vi "CreateIlluminationMask.vi"(7 "# Pixels":u16, 8 "error in (no error)":errorcluster, 9 "Image trig index":u16[](array[numeric]), 10 "Time at P_f":u32[](array[numeric]), 11 "Final step, n":u16[](array[numeric])) -> (0 "error out":errorcluster, 1 "Image trig index OUT":u16[](array[numeric]), 2 "Time at P_f 2":u16[](array[numeric]), 3 "Final step OUT":u16[](array[numeric]), 4 "Time at P_f 2D":u16[][](array[numeric]), 5 "Final step 2D":u16[][](array[numeric]))   [LabVIEW 2016]
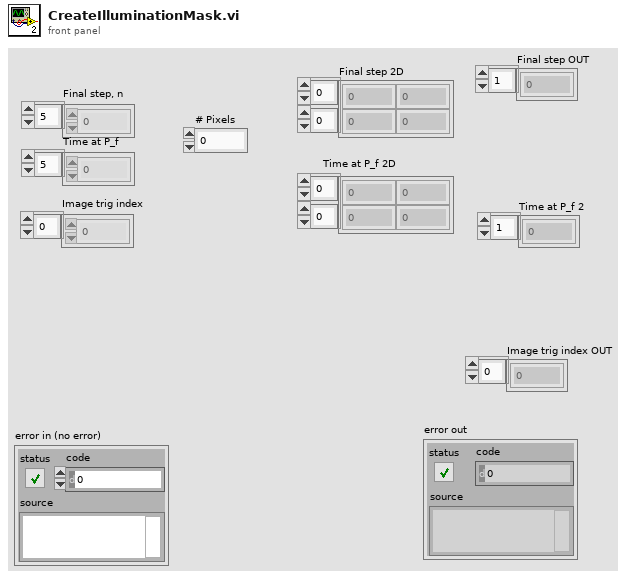
[diagram p1: front panel]
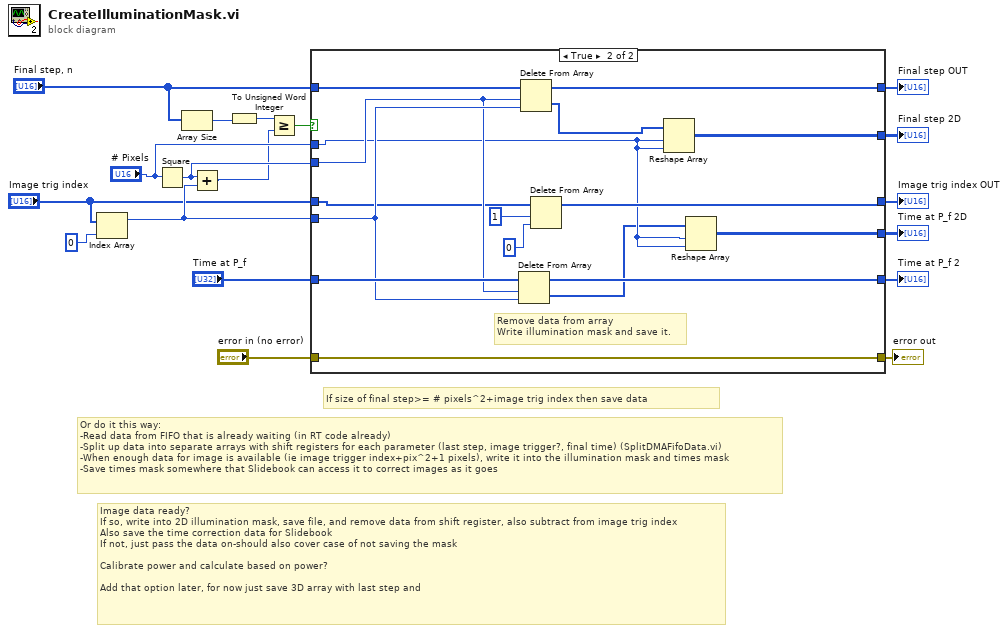
[diagram p0: block diagram]
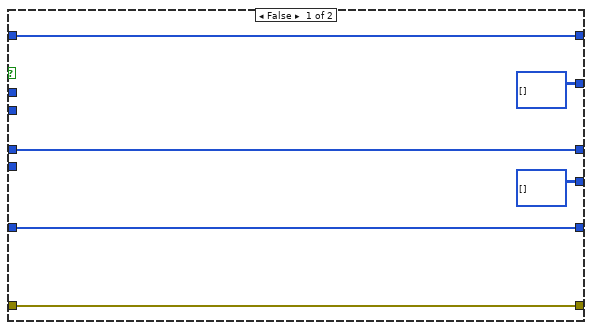
[diagram p2: hidden frame]
diagram:
  # "If size of final step>= # pixels^2+image trig index then save data"
  # "Or do it this way:\n-Read data from FIFO that is already waiting (in RT code already)\n-Split up data into separate arrays with shift registers for each parameter (last step, image trigger?, final time) (SplitDMAFifoData.vi)\n-When enough data for image is available (ie image trigger index+pix^2+1 pixels), write it into the illumination mask and times mask\n-Save times mask somewhere that Slidebook can access it to correct images as it goes"
  # "Image data ready?  \nIf so, write into 2D illumination mask, save file, and remove data from shift register, also subtract from image trig index\nAlso save the time correction data for Slidebook\nIf not, just pass the data on-should also cover case of not saving the mask\n\nCalibrate power and calculate based on power?\n\nAdd that option later, for now just save 3D array with last step and"
  n1 = Index Array(array="Image trig index", index=0) -> (element=w13:u16)
  n2 = Square(x="# Pixels") -> (x^2=w10:u16)
  n3 = Array Size(array="Final step, n") -> (size(s)=w17:i32)
  n4 = Add(x=w10, y=w13) -> (x+y=w1:u16)
  n5 = To Unsigned Word Integer(number=w17) -> (unsigned 16bit integer=w16:u16)
  n6 = Greater Or Equal?(x=w16, y=w1) -> (x >= y?=w15:bool)
  n7 = case shown="True" w15 {
    tunnel: "Final step, n" -> [w23 w39]
    tunnel: w13 -> [_ w35]
    tunnel: "error in (no error)" -> [w24 w40]
    tunnel: "Time at P_f" -> [w21 w37]
    tunnel: w10 -> [_ w34]
    tunnel: [w24 w40] -> w9
    tunnel: [w23 w38] -> w7
    tunnel: "Image trig index" -> [w22 w33]
    tunnel: [w22 w30] -> w4
    tunnel: [w21 w36] -> w2
    tunnel: "# Pixels" -> [_ w27]
    tunnel: [u16[][] [] ("Final step, n") w28] -> w5
    tunnel: [u16[][] [] ("Time at P_f") w26] -> w3
    frame False {
    }
    frame True {
      # "Remove data from array\nWrite illumination mask and save it."
      n8 = Delete From Array(array=w37, length=w34, index=w35) -> (deleted portion=w25:u32[], array with subset deleted=w36:u32[])
      n9 = Delete From Array(array=w39, length=w34, index=w35) -> (deleted portion=w29:u16[], array with subset deleted=w38:u16[])
      n10 = Delete From Array(array=w33, length=1, index=0) -> (array with subset deleted=w30:u16[])  [unwired: 1 out]
      n11 = Reshape Array(w29, w27, w27) -> (w28:u16[][])
      n12 = Reshape Array(w25, w27, w27) -> (w26:u32[][])
    }
  }
  "error out" <- w9
  "Final step OUT" <- w7
  "Final step 2D" <- w5
  "Image trig index OUT" <- w4
  "Time at P_f 2D" <- w3
  "Time at P_f 2" <- w2
